vi "Curve Fit.vi"(0 "Reference (Array)":dbl[](array[numeric]), 5 "Reference (Value)":dbl, 7 "Voltage (Array)":dbl[](array[numeric]), 9 "Voltage (Value)":dbl, 11 "Error In":errorcluster, 12 "index":i32) -> (4 "Slope":dbl, 6 "Intercept":dbl, 8 "Reference Out":dbl[](array[numeric]), 10 "Voltage Out":dbl[](array[numeric]), 15 "Error Out":errorcluster)   [LabVIEW 2019, in "SubVIs.lvlib"]
uses:
  SubVIs.lvlib
  <vilib>/Analysis/NI_AALPro.lvlib
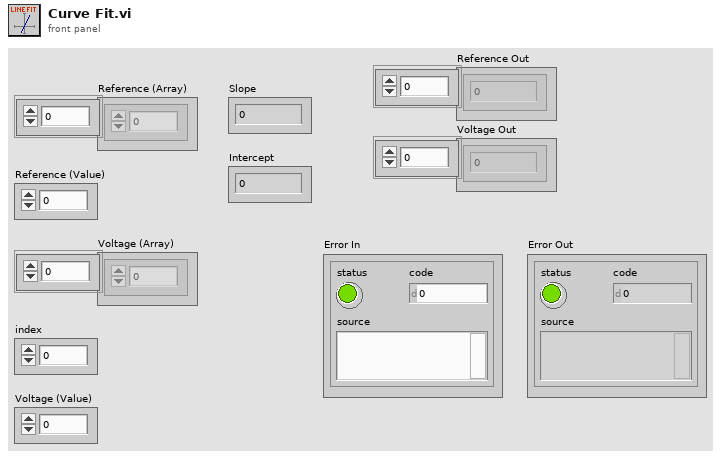
[diagram p1: front panel]
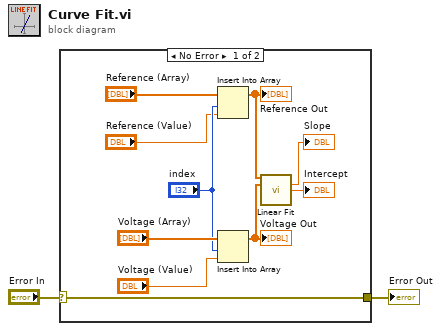
[diagram p0: block diagram]
diagram:
  n1 = case shown="No Error" "Error In" {
    selector: "Error In" -> [w5 w13]
    tunnel: [w5 w13] -> w1
    frame No Error {
      n2 = Insert Into Array(array="Reference (Array)", index="index", new element="Reference (Value)") -> (w4:dbl[])
      "Reference Out" <- w4
      n3 = Insert Into Array(array="Voltage (Array)", index="index", new element="Voltage (Value)") -> (w3:dbl[])
      "Voltage Out" <- w3
      n4 = call <vilib>:"Linear Fit.vi"("Y"=w4, "X"=w3) -> ("slope"=→"Slope":dbl, "intercept"=→"Intercept":dbl)  [unwired: 9 in, 3 out]
    }
    frame Error {
    }
  }
  "Error Out" <- w1
